vi "Set Main Page Monitor Log Directory.vi"(8 "error in":errorcluster, 10 "Monitor Log Directory":string, 11 "Main Page Ref in":T1 format="%.0x") -> (0 "error out":errorcluster, 3 "Main Page Ref out":T1 format="%.0x")   [LabVIEW 2020, in "AIM ARINC 664 Scripting.lvlib"]
uses:
  AIM ARINC 664 Scripting.lvlib
  <vilib>/NI VeriStand/Custom Device API/Custom Device API.lvlib
  Constants.vi
  <vilib>/NI VeriStand/Custom Device API/Set Item Property (String).vi
  <vilib>/NI VeriStand/Custom Device API/Custom Device Item Ref.ctl
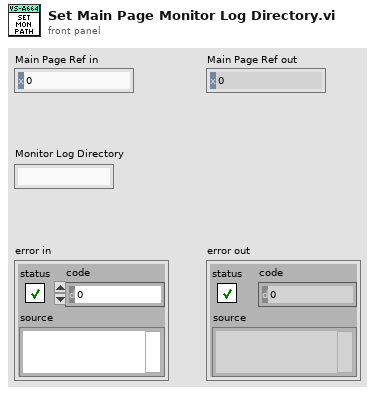
[diagram p1: front panel]
types:
  T1 = typedef "Custom Device API.lvlib/Custom Device Item Ref.ctl" = u64
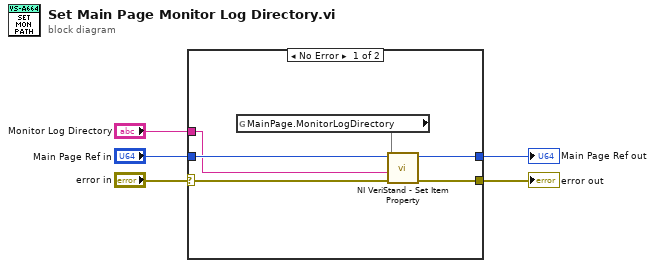
[diagram p0: block diagram]
diagram:
  n1 = case shown="No Error" "error in" {
    selector: "error in" -> [w7 w13]
    tunnel: "Main Page Ref in" -> [w8 w12]
    tunnel: [w11 w13] -> w4
    tunnel: "Monitor Log Directory" -> [w6 _]
    tunnel: [w10 w12] -> w2
    frame No Error {
      n2 = global read "Constants.vi" "MainPage.MonitorLogDirectory"() -> (w9)
      n3 = call-poly <vilib>:"NI VeriStand - Set Item Property.vi"("error in (no error)"=w7, "Value"=w6, "Property Name"=w9, "Item Ref in"=w8) -> ("error out"=w11:errorcluster, "Item Ref out"=w10:T1)  [unwired: 5 in, 1 out]
    }
    frame Error {
    }
  }
  "error out" <- w4
  "Main Page Ref out" <- w2
